vi "sirah_shg.vi"(4 "fcu1_motor, f(x)":string="-2.5795690E+01 * x^2 + 2.0944266E+04 * x - 3.5334445E+06", 5 "lower limit":dbl=320.0 format="%#_13g", 6 "resonator_motor, f(x)":string="-1.33582132E+01 * x^2  + 1.06368361E+03 * x  + 1.59584766E+06", 7 "upper limit":dbl=360.0 format="%#_13g", 8 "error in (no error)":errorcluster, 10 "wavelength (nm)":dbl=327.837 format="%#_16g") -> (0 "error out":errorcluster, 1 "fundamental (nm)":dbl=655.0001186261217 format="%.4f", 2 "value out":dbl=327.5 format="%#_16p")   [LabVIEW 2017]
uses:
  hardware/sirah/sirah.lvlib
panel:
  out "resonator":i32=511452
  out "fcu1":i32=559054
  in  "fcu_offset":i32
  # "November 2018 (pyridine 1)\n\nResonator:\n-2.10126553E+01 * x^2  + 6.31242686E+03 * x + 6.95582109E+05\n\nFCU:\n-6.90079891 * x^2 + 7.69021655E+03 * x - 1.21943926E+06"
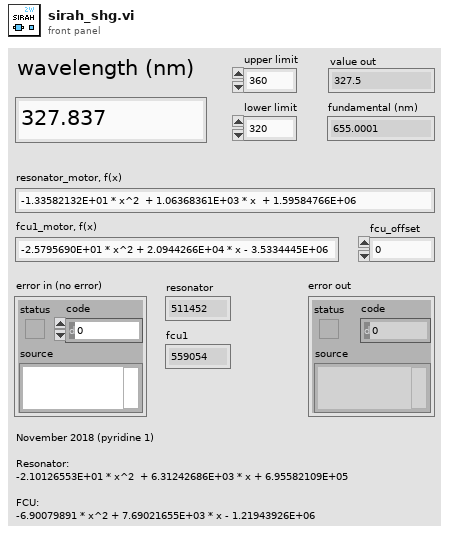
[diagram p1: front panel]
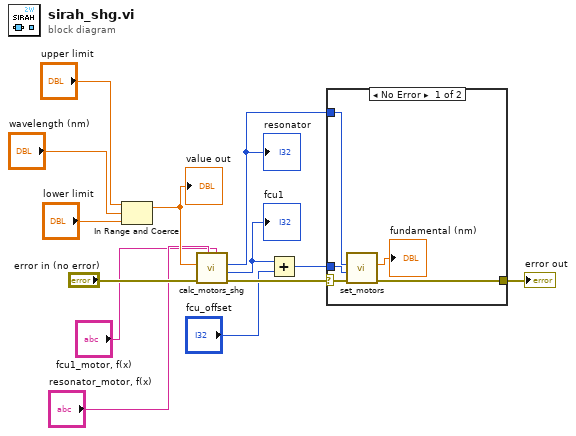
[diagram p0: block diagram]
diagram:
  n1 = In Range and Coerce(upper limit="upper limit", x="wavelength (nm)", lower limit="lower limit") -> (coerced(x)=w6:dbl)  [unwired: 1 out]
  "value out" <- w6
  n2 = call "calc_motors_shg.vi"("fcu1_motor, f(x)"="fcu1_motor, f(x)", "resonator_motor, f(x)"="resonator_motor, f(x)", "error in (no error)"="error in (no error)", "wavelength (nm)"=w6) -> ("error out"=w11:errorcluster, "fcu1"=w3:i32, "resonator"=w10:i32)  [unwired: 5 in]
  "fcu1" <- w3
  "resonator" <- w10
  n3 = Add(x=w3, y="fcu_offset") -> (x+y=w1:i32)
  n4 = case shown="No Error" w11 {
    selector: w11 -> [w18 w19]
    tunnel: [w17 w19] -> w13
    tunnel: w10 -> [w16 _]
    tunnel: w1 -> [w15 _]
    frame No Error {
      n5 = call "set_motors.vi"("error in (no error)"=w18, "SHG"=w15, "resonator"=w16) -> ("error out"=w17:errorcluster, "fundamental (nm)"=→"fundamental (nm)":dbl)  [unwired: 7 in]
    }
    frame Error {
    }
  }
  "error out" <- w13
